vi "Post-Install Custom Action.vi"(10 "Variant":variant) -> (0 "error out":errorcluster)   [LabVIEW 2018]
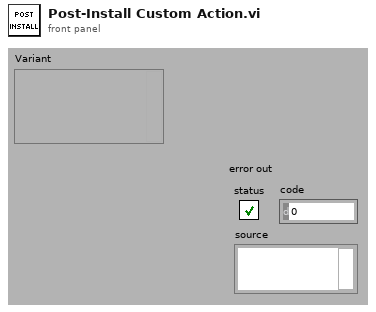
[diagram p1: front panel]
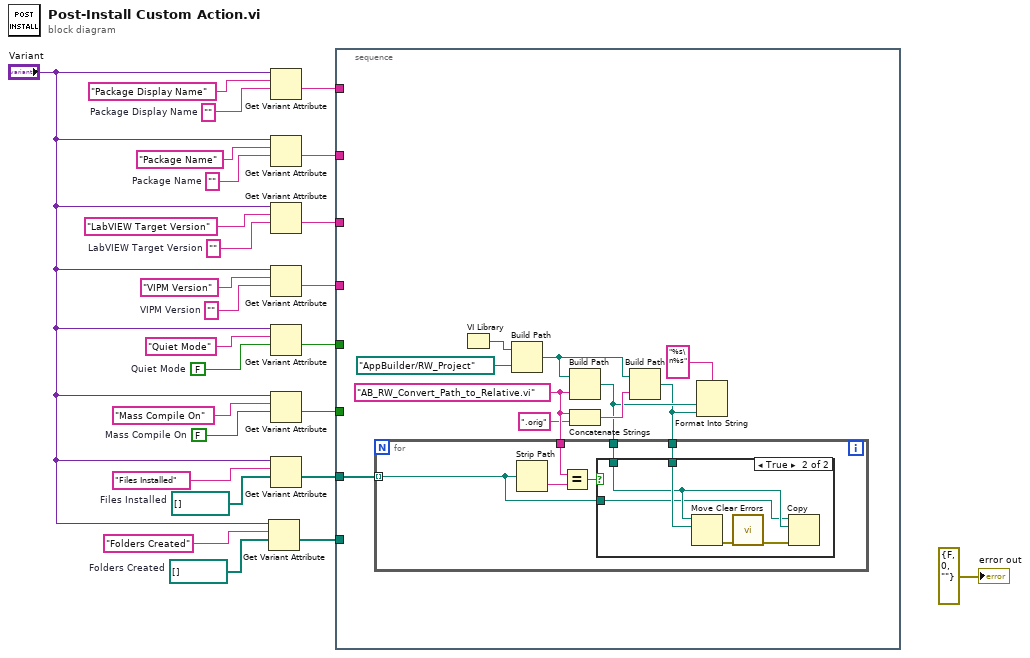
[diagram p0: block diagram]
diagram:
  w1 = path[] []  # Folders Created
  w2 = path[] []  # Files Installed
  w8 = FALSE  # Mass Compile On
  w9 = ""  # Package Display Name
  w16 = FALSE  # Quiet Mode
  w19 = ""  # VIPM Version
  w21 = ""  # LabVIEW Target Version
  w23 = ""  # Package Name
  n1 = Get Variant Attribute(Variant="Variant", name="Folders Created", default value (empty Variant)=w1) -> (value=w6:path[])  [unwired: 1 in, 3 out]
  n2 = Get Variant Attribute(Variant="Variant", name="Package Display Name", default value (empty Variant)=w9) -> (value=w15:string)  [unwired: 1 in, 3 out]
  n3 = Get Variant Attribute(Variant="Variant", name="Package Name", default value (empty Variant)=w23) -> (value=w14:string)  [unwired: 1 in, 3 out]
  n4 = Get Variant Attribute(Variant="Variant", name="LabVIEW Target Version", default value (empty Variant)=w21) -> (value=w13:string)  [unwired: 1 in, 3 out]
  n5 = Get Variant Attribute(Variant="Variant", name="VIPM Version", default value (empty Variant)=w19) -> (value=w12:string)  [unwired: 1 in, 3 out]
  n6 = Get Variant Attribute(Variant="Variant", name="Quiet Mode", default value (empty Variant)=w16) -> (value=w11:bool)  [unwired: 1 in, 3 out]
  n7 = Get Variant Attribute(Variant="Variant", name="Mass Compile On", default value (empty Variant)=w8) -> (value=w10:bool)  [unwired: 1 in, 3 out]
  n8 = Get Variant Attribute(Variant="Variant", name="Files Installed", default value (empty Variant)=w2) -> (value=w5:path[])  [unwired: 1 in, 3 out]
  n9 = stacked-sequence {
    tunnel: w15 -> [_]
    tunnel: w14 -> [_]
    tunnel: w13 -> [_]
    tunnel: w12 -> [_]
    tunnel: w11 -> [_]
    tunnel: w10 -> [_]
    tunnel: w5 -> [w27]
    tunnel: w6 -> [_]
    frame #0 {
      w34 = "AB_RW_Convert_Path_to_Relative.vi"
      n10 = VI Library() -> (path=w36:path)
      n11 = Build Path(base path=w36, name or relative path=path "AppBuilder/RW_Project") -> (appended path=w32:path)
      n12 = Build Path(base path=w32, name or relative path=w34) -> (appended path=w30:path)
      n13 = Concatenate Strings(w34, ".orig" ("string")) -> (w31:string)
      n14 = Build Path(base path=w32, name or relative path=w31) -> (appended path=w29:path)
      n15 = for {
        tunnel: w27 -> [w39] mode=indexing
        tunnel: w34 -> [w40]
        tunnel: w30 -> [w38]
        tunnel: w29 -> [w37]
        n16 = Strip Path(path=w39) -> (name=w41:string)  [unwired: 1 out]
        n17 = Equal?(x=w40, y=w41) -> (x = y?=w42:bool)
        n18 = case shown="True" w42 {
          tunnel: w39 -> [_ w43]
          tunnel: w38 -> [_ w44]
          tunnel: w37 -> [_ w47]
          frame False {
          }
          frame True {
            n19 = Move(source path=w44, 10:w47) -> (error out=w46:errorcluster)  [unwired: 3 in, 2 out]
            n20 = call <vilib>:"Clear Errors.vi"("error in (no error)"=w46) -> ("error out"=w45:errorcluster)  [unwired: 5 in, 1 out]
            n21 = Copy(8:w45, 10:w44, 11:w43) -> ()  [unwired: 2 in, 3 out]
          }
        }
      }
      n22 = Format Into String(format string="%s\n%s", w30, w29) -> ()  [unwired: 2 in, 2 out]
    }
  }
  "error out" <- errorcluster {"status"=FALSE, "code"=0, "source"=""} ("error out")
